vi "Test Pure Mock Pass if Expected API Call Made Asynchronously.vi"(8 "error in (no error)":errorcluster, 11 "Test Case In":refnum<class "Responsive Mock Expectation Test.lvclass">) -> (0 "error out":errorcluster, 3 "Test Case Out":refnum<class "Responsive Mock Expectation Test.lvclass">)   [LabVIEW 2020, in "Responsive Mock Expectation Test.lvclass"]
uses:
  Responsive Mock Expectation Test.lvclass
  Responsive Mock Expectation Test.lvclass/Responsive Mock Expectation Test.ctl
  source/Expectations/One/One.lvclass
  Test Doubles/Test Interface Pure Mock/Test Interface Pure Mock.lvclass
  C:/git/astemes-lmock/source/Framework/Pure Mock/Pure Mock.lvclass
  C:/git/astemes-lmock/source/Core/Mock/Mock.lvclass
  C:/git/astemes-lmock/tests/Test Doubles/Test Interface Pure Mock/Test Interface Pure Mock.lvclass
  C:/git/astemes-lmock/tests/Test Doubles/Test Interface/Test Interface.lvclass
  C:/Program Files (x86)/National Instruments/LabVIEW 2020/vi.lib/Astemes/LUnit/Test Case.lvclass
  C:/Program Files (x86)/National Instruments/LabVIEW 2020/vi.lib/Astemes/LUnit/LUnit Runnable.lvclass
  C:/git/astemes-lmock/tests/Expectation Test/Responsive Mock Expectation Test.lvclass
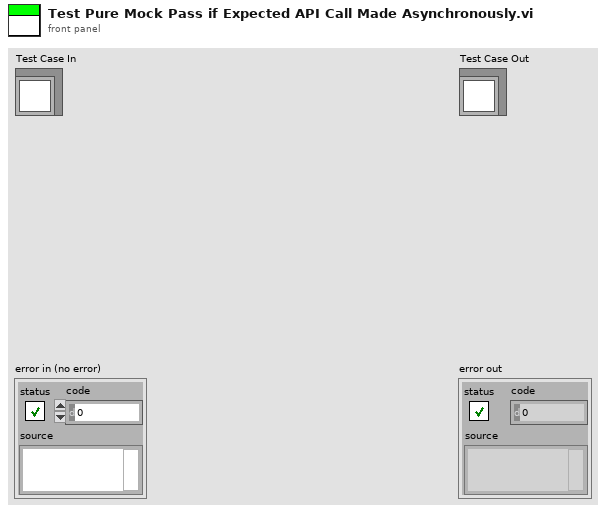
[diagram p1: front panel]
types:
  T1 = enum16{"", "Passed", "Failed", "Error", "Skipped", "Setup Error", "Broken", "Teardown Error"}
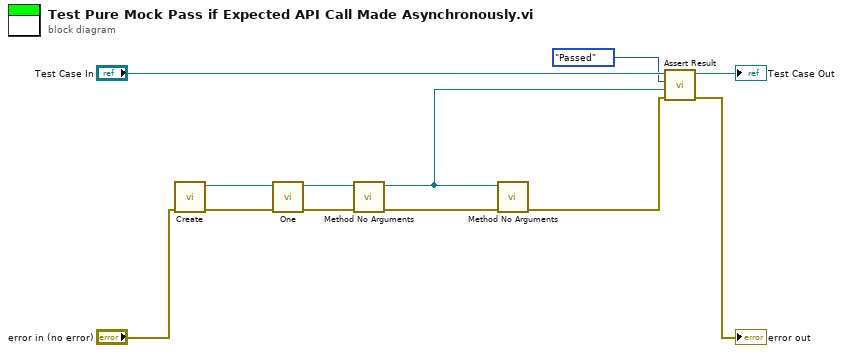
[diagram p0: block diagram]
diagram:
  n1 = call "Create.vi"("error in (no error)"="error in (no error)") -> ("error out"=w11:errorcluster, "Test Interface Mock Out"=w12:refnum<class "Test Interface Pure Mock.lvclass">)  [unwired: 9 in]
  n2 = call "One.vi"("error in (no error)"=w11, "Mock in"=w12) -> ("error out"=w9:errorcluster, "Mock out"=w10:refnum<class "Test Interface Pure Mock.lvclass">)  [unwired: 8 in]
  n3 = call-dynamic "Method No Arguments.vi"("error in (no error)"=w9, "Mock In"=w10) -> ("error out"=w8:errorcluster, "Mock Out"=w1:refnum<class "Test Interface Pure Mock.lvclass">)  [unwired: 8 in]
  n4 = call-dynamic "Method No Arguments.vi"("error in (no error)"=w8, "Mock In"=w1) -> ("error out"=w2:errorcluster)  [unwired: 8 in, 1 out]
  n5 = call "Assert Result.vi"("error in (no error)"=w2, "Mock"=w1, "Status"=T1."Passed", "LUnit Test Case In"="Test Case In") -> ("error out"=→"error out":errorcluster, "LUnit Test Case Out"=→"Test Case Out":refnum<class "Responsive Mock Expectation Test.lvclass">)  [unwired: 6 in]
